vi "Part 1.vi"(11 "Input":string) -> (3 "Output":i64)   [LabVIEW 2021]
panel:
  out "Unknowns scanners left":i32
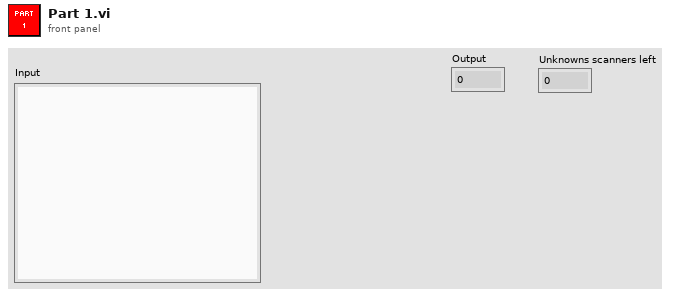
[diagram p1: front panel]
types:
  T1 = cluster{"Beacons":cluster{"X":i64, "Y":i64, "Z":i64}[]}[]
  T2 = cluster{"Beacons":cluster{"X":i64, "Y":i64, "Z":i64}[]}
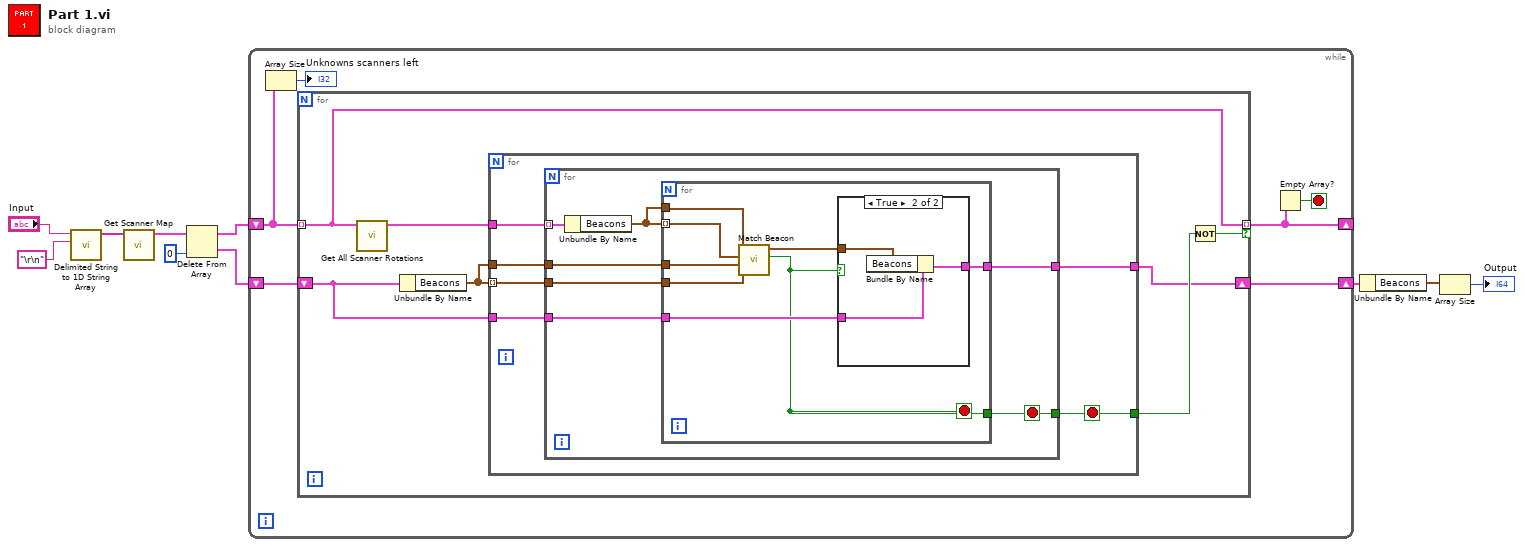
[diagram p0: block diagram]
diagram:
  n1 = call <vilib>:"Delimited String to 1D String Array.vi"("delimiter"="\r\n", "delimited string"="Input") -> ("string array"=w8:string[])  [unwired: 9 in]
  n2 = call "Get Scanner Map.vi"("Input"=w8) -> ("Scanners"=w5:T1)  [unwired: 10 in]
  n3 = Delete From Array(array=w5, index=0) -> (deleted portion=w3:T2, array with subset deleted=w4:T1)  [unwired: 1 in]
  n4 = while {
    shift-right: [w15] -> w6
    shift-left: w3 -> [w16]
    shift-right: [w14] -> _
    shift-left: w4 -> [w12]
    stop <- w13 stop-if-true
    n5 = Array Size(array=w12) -> (size(s)=→"Unknowns scanners left":i32)
    n6 = for {
      tunnel: w12 -> [w22] mode=indexing
      shift-right: [w18] -> w15
      shift-left: w16 -> [w17]
      tunnel: [w22] -> w14 mode=indexing if=w23
      n7 = call "Get All Scanner Rotations.vi"("Scanner"=w22) -> ("Scanner Rotations"=w21:T1)  [unwired: 10 in]
      n8 = Unbundle By Name(w17) -> ("Beacons"=w19:cluster{"X":i64, "Y":i64, "Z":i64}[])
      n9 = for {
        tunnel: [w29] -> w20
        tunnel: w21 -> [w27]
        tunnel: w19 -> [w28] mode=indexing
        tunnel: w19 -> [w26]
        tunnel: [w25] -> w18
        tunnel: w17 -> [w24]
        stop <- w29 stop-if-true
        n10 = for {
          tunnel: [w31] -> w29
          tunnel: w28 -> [w36]
          tunnel: w27 -> [w33] mode=indexing
          tunnel: w26 -> [w34]
          tunnel: [w32] -> w25
          tunnel: w24 -> [w30]
          stop <- w31 stop-if-true
          n11 = Unbundle By Name(w33) -> ("Beacons"=w35:cluster{"X":i64, "Y":i64, "Z":i64}[])
          n12 = for {
            tunnel: w36 -> [w39]
            tunnel: w35 -> [w41] mode=indexing
            tunnel: w35 -> [w42]
            tunnel: w34 -> [w40]
            tunnel: w30 -> [w43]
            tunnel: [w44] -> w32
            tunnel: [w37] -> w31
            stop <- w37 stop-if-true
            n13 = call "Match Beacon.vi"("Known Beacon"=w39, "Known Beacons"=w40, "Unknown Beacon"=w41, "Unknown Beacons"=w42) -> ("Match?"=w37:bool, "New Beacons"=w38:cluster{"X":i64, "Y":i64, "Z":i64}[])  [unwired: 6 in]
            n14 = case shown="True" w37 {
              tunnel: [w45 w47] -> w44
              tunnel: w43 -> [w45 w48]
              tunnel: w38 -> [_ w46]
              frame False {
              }
              frame True {
                n15 = Bundle By Name(cluster=w48, "Beacons"=w46) -> (w47:T2)
              }
            }
          }
        }
      }
      n16 = Not(x=w20) -> (.not. x?=w23:bool)
    }
    n17 = Empty Array?(array=w14) -> (empty?=w13:bool)
  }
  n18 = Unbundle By Name(w6) -> ("Beacons"=w2:cluster{"X":i64, "Y":i64, "Z":i64}[])
  n19 = Array Size(array=w2) -> (size(s)=→"Output":i32)
